vi "Create Server Configuration File.vi"(8 "error in (no error)":errorcluster, 10 "sshd_config":string, 11 "Server Fixture in":refnum<class "Server Fixture.lvclass">) -> (0 "error out":errorcluster, 3 "Server Fixture out":refnum<class "Server Fixture.lvclass">)   [LabVIEW 2013, in "libssh2_integration_tests.lvlib" / "Server Fixture.lvclass"]
uses:
  Server Fixture.lvclass
  Server Fixture.lvclass/Server Fixture.ctl
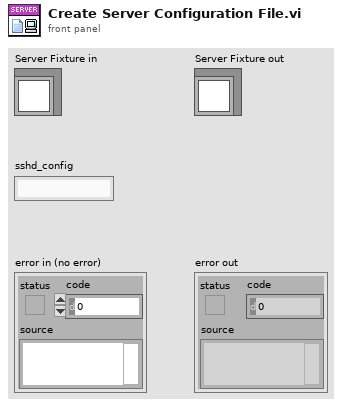
[diagram p1: front panel]
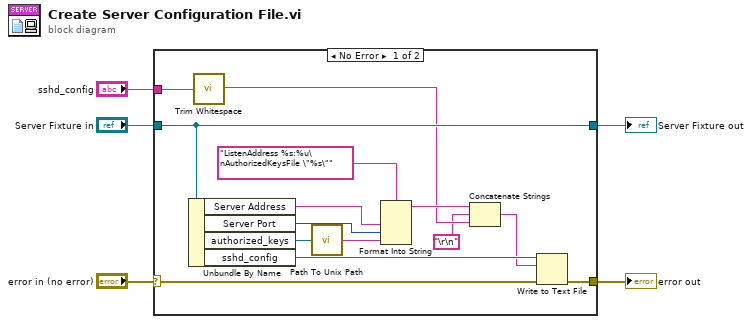
[diagram p0: block diagram]
diagram:
  n1 = case shown="No Error" "error in (no error)" {
    selector: "error in (no error)" -> [w14 w21]
    tunnel: [w13 w21] -> w4
    tunnel: [w15 w20] -> w2
    tunnel: "Server Fixture in" -> [w15 w20]
    tunnel: "sshd_config" -> [w9 _]
    frame No Error {
      n2 = Unbundle By Name(w15) -> ("Server Address"=w11:string, "Server Port"=w12:u16, "authorized_keys"=w17:path, "sshd_config"=w16:path)
      n3 = call <vilib>:"Trim Whitespace.vi"("string"=w9) -> ("trimmed string"=w8:string)  [unwired: 1 in]
      n4 = call "Path To Unix Path.vi"("path"=w17) -> ("unix path"=w18:string)  [unwired: 1 in]
      n5 = Format Into String(format string="ListenAddress %s:%u\nAuthorizedKeysFile \"%s\"" ("sshd_config"), w11, w12, w18) -> (resulting string=w10:string)  [unwired: 2 in, 1 out]
      n6 = Concatenate Strings(w10, "\r\n", w8) -> (w7:string)
      n7 = Write to Text File(file (use dialog)=w16, text=w7, error in=w14) -> (error out=w13:errorcluster)  [unwired: 1 in, 2 out]
    }
    frame Error {
    }
  }
  "error out" <- w4
  "Server Fixture out" <- w2
